vi "Controller - Get Axis Parameters (subVI).vi"(8 "Axis":i16, 9 "Axis Parameters":string[](array[string]), 10 "error in (no error)":errorcluster, 11 "Automation Refnum in":refnum<k7>) -> (1 "Axis Parameter Values":dbl[](array[numeric]), 2 "error out":errorcluster, 3 "Automation Refnum out":refnum<k7>)   [LabVIEW 2020]
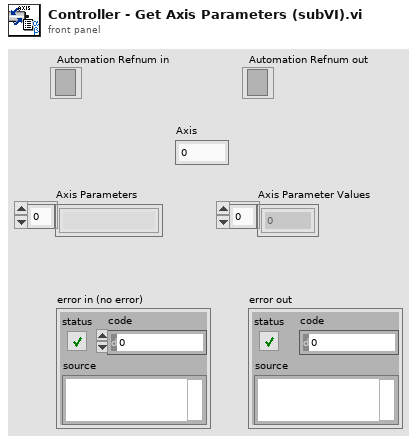
[diagram p1: front panel]
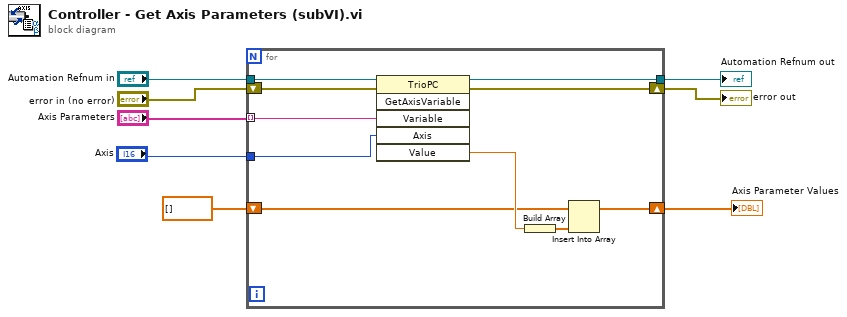
[diagram p0: block diagram]
diagram:
  n1 = for {
    shift-right: [w16] -> w1
    shift-left: dbl[] [] ("Array") -> [w15]
    tunnel: "Automation Refnum in" -> [w14]
    tunnel: "Axis Parameters" -> [w13] mode=indexing
    tunnel: "Axis" -> [w12]
    tunnel: [w11] -> w4
    shift-right: [w10] -> w3
    shift-left: "error in (no error)" -> [w9]
    n2 = invoke class="TrioPC" method="GetAxisVariable"(reference=w14, error in=w9, "Variable"=w13, "Axis"=w12) -> (reference out=w11:refnum<k7>, error out=w10:errorcluster, "Value"=w18:dbl)  [unwired: 2 in, 3 out]
    n3 = Build Array(w18) -> (w17:dbl[])
    n4 = Insert Into Array(array=w15, new element=w17) -> (w16:dbl[])  [unwired: 1 in]
  }
  "error out" <- w3
  "Automation Refnum out" <- w4
  "Axis Parameter Values" <- w1
